vi "draw waveform 3.vi"() -> ()   [LabVIEW 2009]
panel:
  in  "Clear all points":bool
  in  "balance parameter":dbl(slide)=-1.0 scale=-0.1..1.0
  in  "Auto-update waveform":bool
  in  "stop [esc]":bool
  in  "Delete point [F2]":bool
  in  "discrete points":cluster{"time":dbl, "value":dbl}[](array[cluster])
  out "XY Graph":cluster{dbl[], "Best Cubic Spline Fit":dbl[]}(graph)
  # "time"
  # "value"
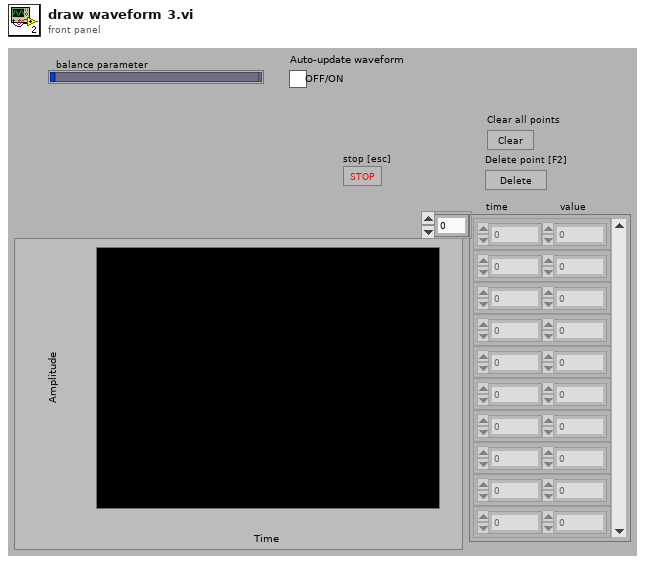
[diagram p1: front panel]
types:
  T1 = typedef "LVPoint32TypeDef.ctl" = cluster{"Horizontal":i32, "Vertical":i32}
  T2 = typedef "LVPositionTypeDef.ctl" = cluster{"Left":i32, "Top":i32}
  T3 = cluster{"XScale.Minimum":dbl, "X Scale.Range:Minimum":dbl}[]
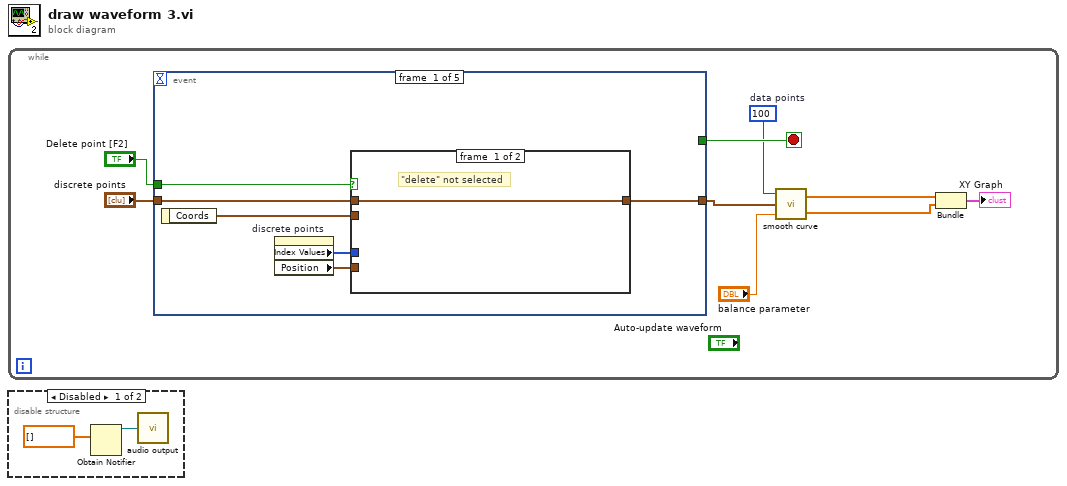
[diagram p0: block diagram]
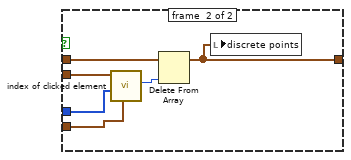
[diagram p3: hidden frame]
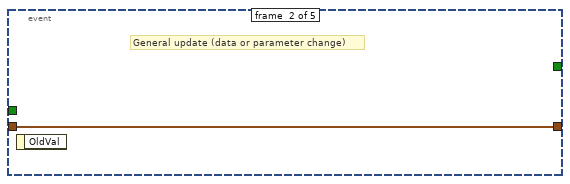
[diagram p4: hidden frame]
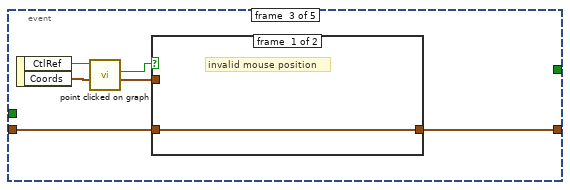
[diagram p5: hidden frame]
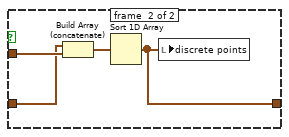
[diagram p6: hidden frame]
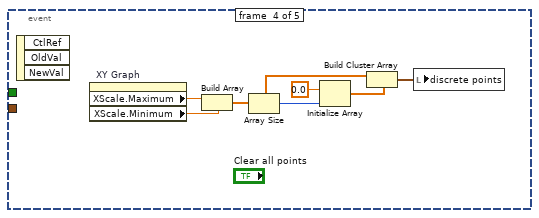
[diagram p7: hidden frame]
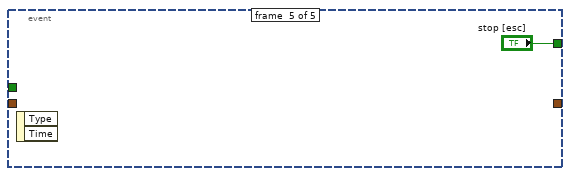
[diagram p8: hidden frame]
diagram:
  n1 = while {
    stop <- w9 stop-if-true
    w1 = 100  # data points
    n2 = event shown="[2] \"XY Graph\": Mouse Down" {
      selector: _ -> [_ _ _ _ _]
      dyn-events: _ -> [_ _ _ _ _]
      timeout: _ -> [_ _ _ _ _]
      tunnel: [_ _ _ _ "stop [esc]"] -> w9
      tunnel: "Delete point [F2]" -> [w13 _ _ _ _]
      tunnel: "discrete points" -> [w11 w23 w27 _ _]
      tunnel: [w10 w23 w24 _ _] -> w6
      event #0 {
        n3 = event-data() -> ("Coords"=w14:T1)  [unwired: 1 in]
        n4 = property on="discrete points" class="Arr (strict)"() -> ("Index Values"=w15:u32[], "Position"=w12:T2)  [unwired: 2 in, 2 out]
        n5 = case shown="True" w13 {
          tunnel: w15 -> [_ w22]
          tunnel: w14 -> [_ w21]
          tunnel: w12 -> [_ w19]
          tunnel: w11 -> [w16 w18]
          tunnel: [w16 w17] -> w10
          frame #0 {
            # "\"delete\" not selected"
          }
          frame #1 {
            n6 = call "index of clicked element.vi"("Control cords"=w19, "Index Values"=w22, "Mouse cords"=w21) -> ("element index"=w20:i32)  [unwired: 8 in]
            n7 = Delete From Array(array=w18, index=w20) -> (array with subset deleted=w17:cluster{"time":dbl, "value":dbl}[])  [unwired: 1 in, 1 out]
            n8 = local write "discrete points"(w17) -> ()
          }
        }
      }
      event #1 {
        # "General update (data or parameter change)"
        n9 = event-data() -> ()  [unwired: 1 in, 1 out]
      }
      event #2 {
        n10 = event-data() -> ("CtlRef"=w29:refnum<vi>, "Coords"=w28:T1)  [unwired: 1 in]
        n11 = call "point clicked on graph.vi"("Mouse Position"=w28, "Graphchart reference"=w29) -> ("Point clicked"=w26:cluster{"x":dbl, "y":dbl}, "Valid mouse position"=w25:bool)  [unwired: 8 in]
        n12 = case shown="True" w25 {
          tunnel: w27 -> [w30 w32]
          tunnel: w26 -> [_ w34]
          tunnel: [w30 w31] -> w24
          frame #0 {
            # "invalid mouse position"
          }
          frame #1 {
            n13 = Build Array (concatenate)(w32, w34) -> (w33:cluster{"x":dbl, "y":dbl}[])
            n14 = Sort 1D Array(array=w33) -> (sorted array=w31:cluster{"x":dbl, "y":dbl}[])
            n15 = local write "discrete points"(w31) -> ()
          }
        }
      }
      event #3 {
        n16 = event-data() -> ()  [unwired: 1 in, 3 out]
        n17 = property on="XY Graph" class="XYGraph (strict)"() -> ("XScale.Maximum"=w41:dbl, "XScale.Minimum"=w40:dbl)  [unwired: 2 in, 2 out]
        n18 = Build Array(w41, w40) -> (w39:dbl[])
        n19 = Array Size(array=w39) -> (size(s)=w37:i32)
        n20 = Initialize Array(0.0 ("X Scale.Range:Minimum"), w37) -> (w36:dbl[])
        n21 = Build Cluster Array(w39, w36) -> (w35:T3)
        n22 = local write "discrete points"(w35) -> ()
      }
      event #4 {
        n23 = event-data() -> ()  [unwired: 1 in, 2 out]
      }
    }
    n24 = call "smooth curve.vi"("balance parameter"="balance parameter", "discrete points"=w6, "data points"=w1) -> ("y"=w3:dbl[], "x"=w4:dbl[])
    n25 = Bundle("x"=w4, "y"=w3) -> (→"XY Graph":cluster{"x":dbl[], "y":dbl[]})  [unwired: 1 in]
  }
  n26 = disable-structure shown="Disabled" {
    frame #0 {
      n27 = Obtain Notifier(notification data type=sgl[] []) -> (notifier out=w43:refnum<notifier>)  [unwired: 3 in, 2 out]
      n28 = call "audio output.vi"("notifier"=w43) -> ()
    }
    frame #1 {
    }
  }
